vi "cm2nm_Calculate_Coordinate_transform.vi"(11 "PairedFiducialCoordinates":T3(array[cluster])) -> (1 "C- vector offset -- reference":T1, 2 "B - vector offset":T1, 3 "A - Transformation Matrix":T1)   [LabVIEW 2011]
uses:
  <vilib>/Analysis/Matrix/Datatypes/RealMatrix.ctl
  <vilib>/Analysis/Matrix/NI_Matrix.lvlib
panel:
  out "B - vector offset 2":T1
  out "A - Transformation Matrix 2":T1
  out "output cluster":T2
  out "Array":T3(array[cluster])
  out "Ax + B":T1
  out "error":i32 format="%.3p"
  # "X1 = AX2 + B"
  # "Fiducial Location Pair"
  # "Current Instrument Fiducial Location"
  # "Reference Instrument Fiducial Location"
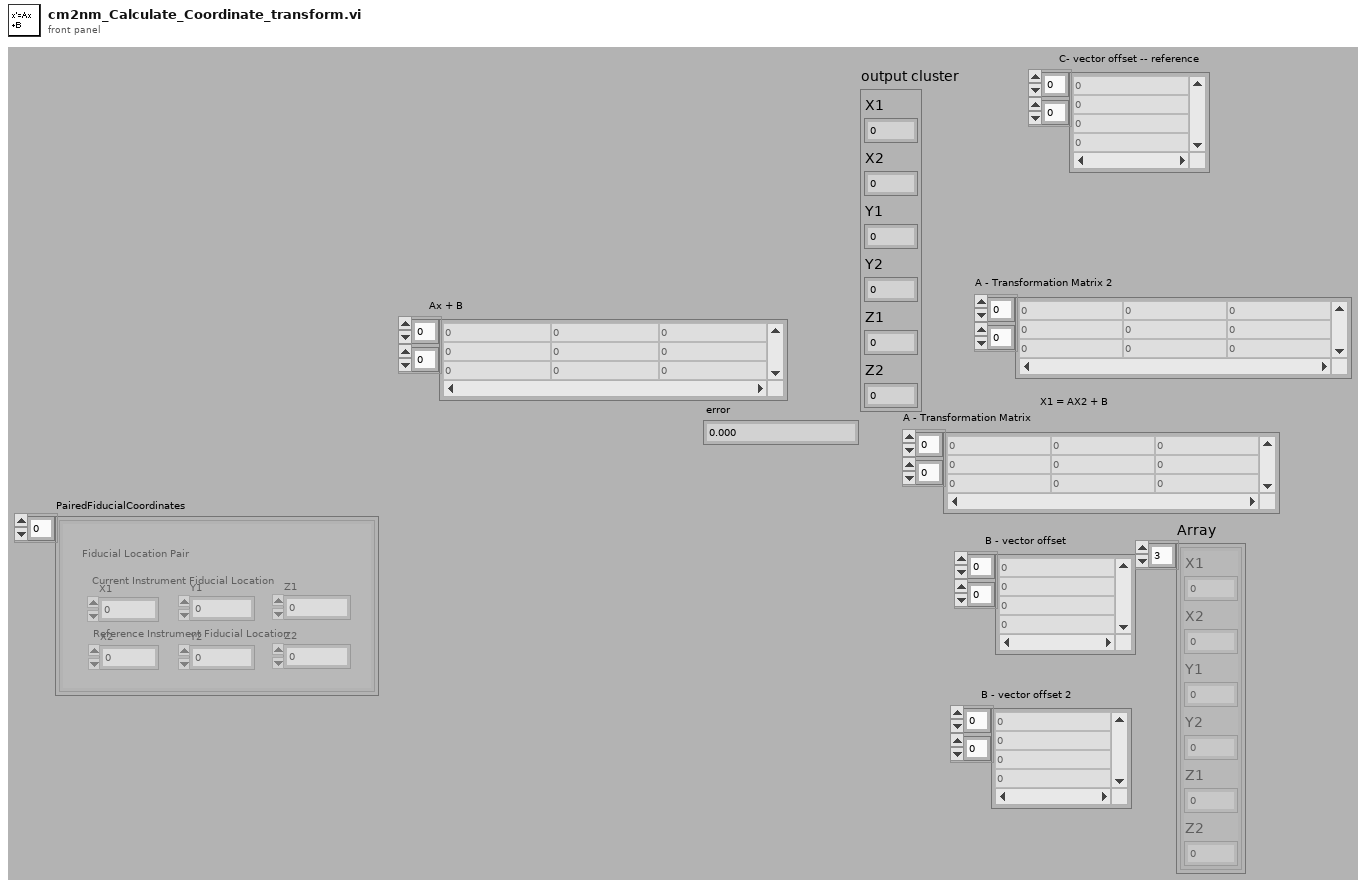
[diagram p1: front panel]
types:
  T1 = typedef "NI_Matrix.lvlib/RealMatrix.ctl" = dbl[][]
  T2 = cluster{"X1":dbl, "X2":dbl, "Y1":dbl, "Y2":dbl, "Z1":dbl, "Z2":dbl}
  T3 = cluster{"X1":dbl, "X2":dbl, "Y1":dbl, "Y2":dbl, "Z1":dbl, "Z2":dbl}[]
  T4 = typedef "Fiducial_pair.ctl" = cluster{"X1":dbl, "X2":dbl, "Y1":dbl, "Y2":dbl, "Z1":dbl, "Z2":dbl}
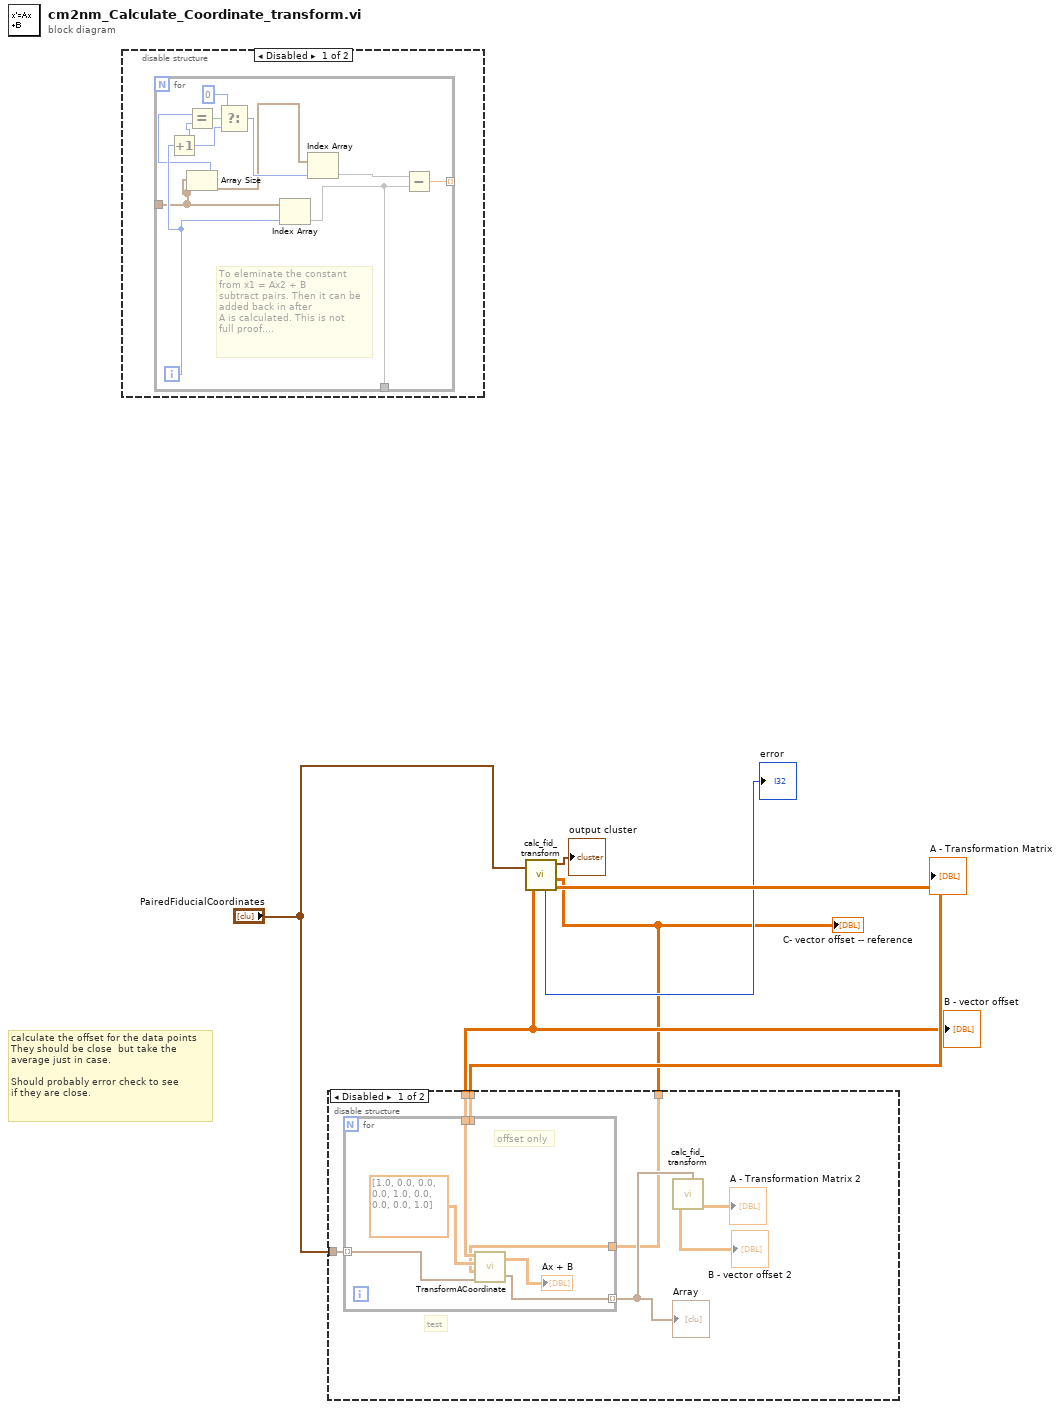
[diagram p0: block diagram]
diagram:
  # "calculate the offset for the data points\nThey should be close  but take the\naverage just in case.\n\nShould probably error check to see\nif they are close."
  n1 = disable-structure shown="Disabled" {
    frame Disabled {
      n2 = for {
        tunnel: _ -> [w10]
        tunnel: [w11] -> _ mode=indexing
        tunnel: [w7] -> _
        i -> [w14]
        # "To eleminate the constant\nfrom x1 = Ax2 + B\nsubtract pairs. Then it can be\nadded back in after\nA is calculated. This is not\nfull proof...."
        n3 = Increment(x=w14) -> (x+1=w8:i32)
        n4 = Array Size(array=w10) -> (size(s)=w9:i32)
        n5 = Equal?(x=w9, y=w8) -> (x = y?=w16:bool)
        n6 = Select(t=0, s=w16, f=w8) -> (s? t:f=w13:i32)
        n7 = Index Array(array=w10, index=w14) -> (element=w7)
        n8 = Index Array(array=w10, index=w13) -> (element=w12)
        n9 = Subtract(x=w12, y=w7) -> (x-y=w11:dbl)
      }
    }
    frame Enabled {
    }
  }
  n10 = call "calc_fid_transform.vi"("PairedFiducialCoordinates"="PairedFiducialCoordinates") -> ("B"=w5:T1, "error"=→"error":i32, "A"=w6:T1, "C"=w1:T1, "ShiftedPairedFiducials"=→"output cluster":T4)  [unwired: 2 in]
  "A - Transformation Matrix" <- w6
  "B - vector offset" <- w5
  "C- vector offset -- reference" <- w1
  n11 = disable-structure shown="Disabled" {
    disable-tunnel: w6 -> [w23 _]
    disable-tunnel: w5 -> [w22 _]
    disable-tunnel: "PairedFiducialCoordinates" -> [w21 _]
    disable-tunnel: w1 -> [w17 _]
    frame Disabled {
      # "test"
      n12 = for {
        tunnel: w23 -> [_]
        tunnel: w22 -> [w26]
        tunnel: [w28] -> w20 mode=indexing
        tunnel: w21 -> [w27] mode=indexing
        tunnel: w17 -> [w24]
        # "offset only"
        n13 = call "TransformACoordinate.vi"("Input"=w27, "C"=w24, "A"=T1 [[1.0, 0.0, 0.0], [0.0, 1.0, 0.0], [0.0, 0.0, 1.0]], "B"=w26) -> ("Result"=w28:T2, "Ax + B"=→"Ax + B":T1)
      }
      "Array" <- w20
      n14 = call "calc_fid_transform.vi"("PairedFiducialCoordinates"=w20) -> ("B"=→"B - vector offset 2":T1, "A"=→"A - Transformation Matrix 2":T1)  [unwired: 2 in, 3 out]
    }
    frame Enabled {
    }
  }
